vi "acquire single wave subvi.vi"(8 "error in (no error)":errorcluster, 10 "read buffer 5":string, 11 "VISA Refnum in":refnum<visa-resource-name>) -> (0 "Enum":enum16{"Idle", "Start"}(ring), 1 "String":string, 2 "read buffer":string, 3 "read buffer 3":string, 4 "Array":i32[](array[numeric]), 5 "read buffer 2":string, 6 "read buffer 6":string, 7 "read buffer 4":string)   [LabVIEW 2013]
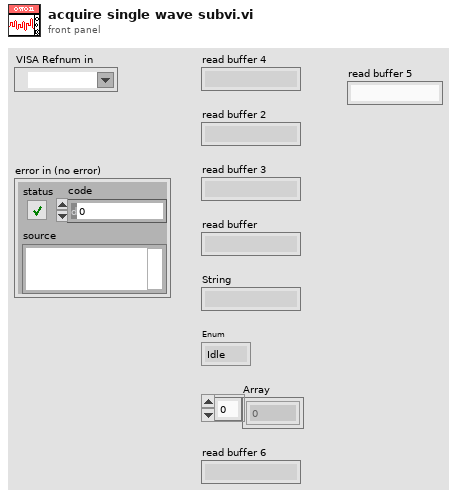
[diagram p1: front panel]
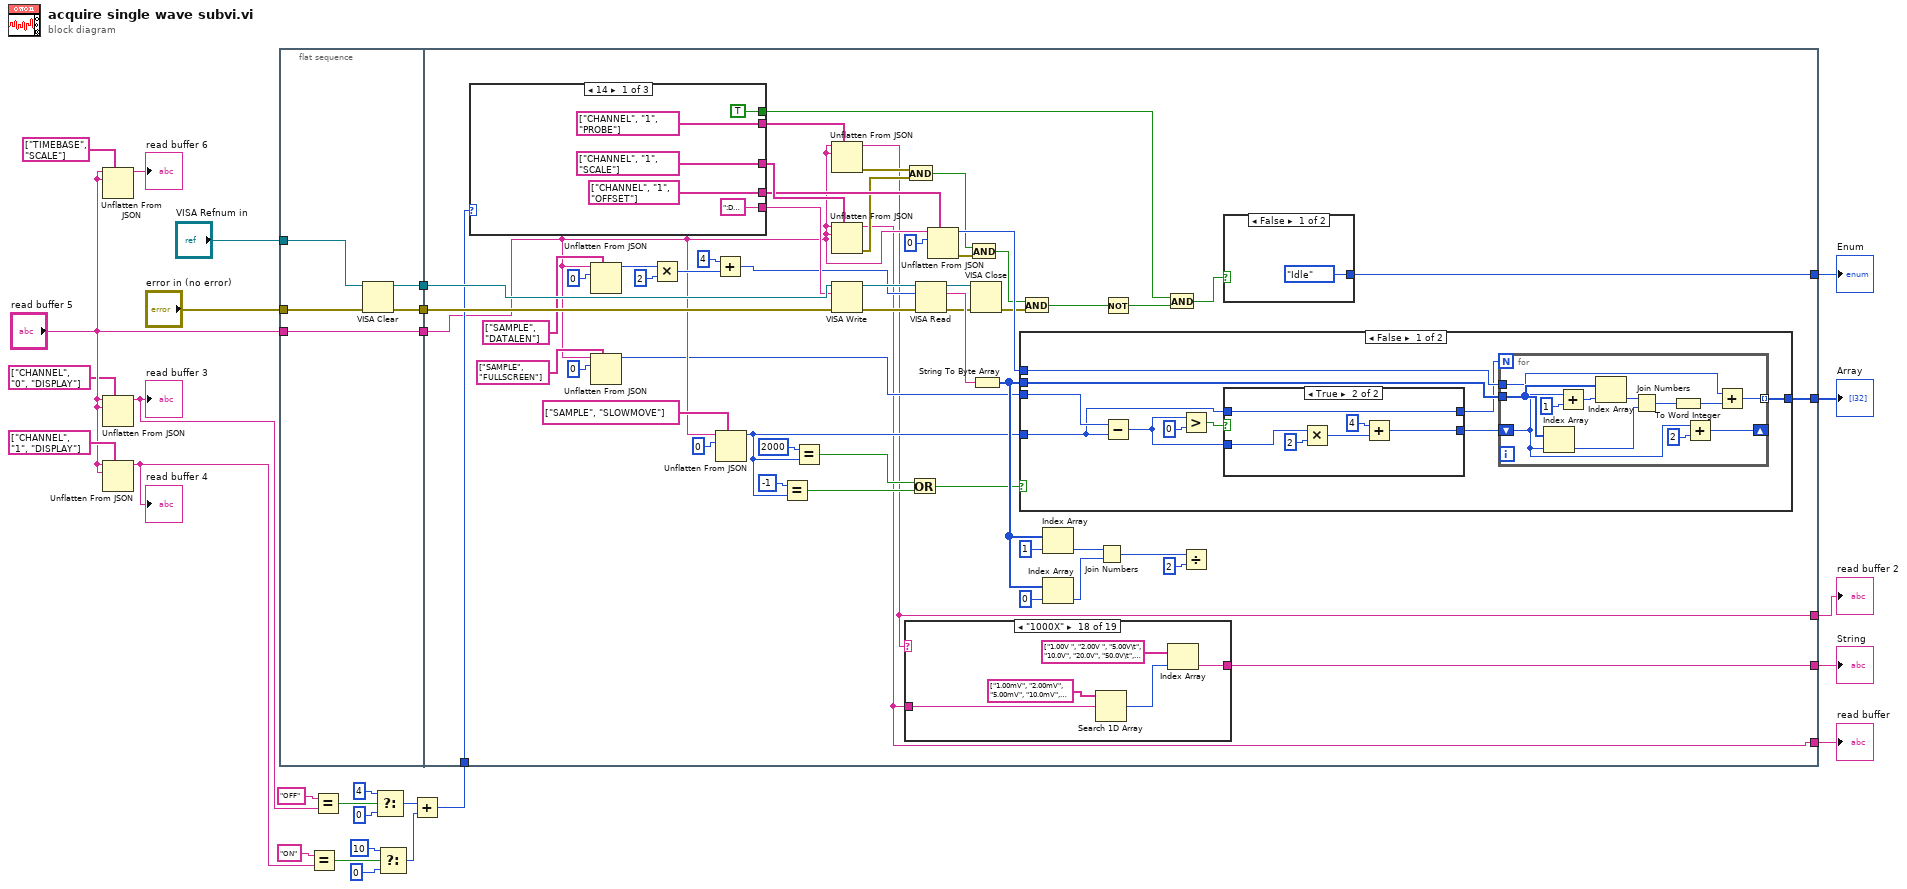
[diagram p0: block diagram]
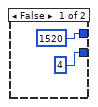
[diagram p2: hidden frame]
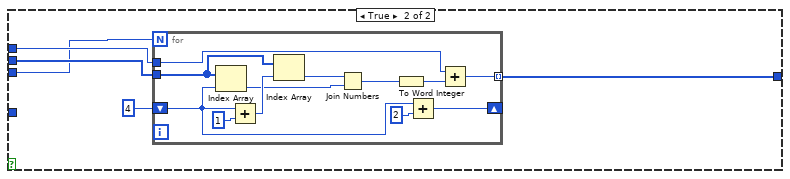
[diagram p3: hidden frame]
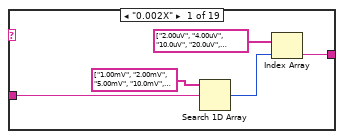
[diagram p4: hidden frame]
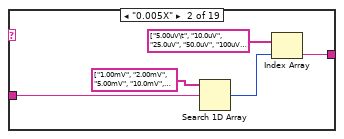
[diagram p5: hidden frame]
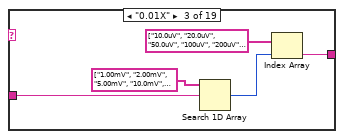
[diagram p6: hidden frame]
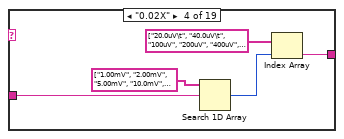
[diagram p7: hidden frame]
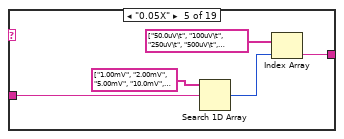
[diagram p8: hidden frame]
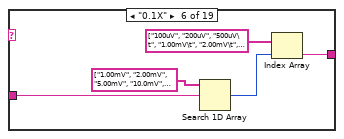
[diagram p9: hidden frame]
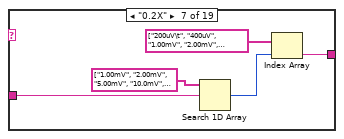
[diagram p10: hidden frame]
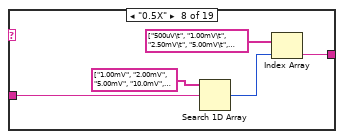
[diagram p11: hidden frame]
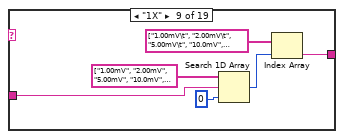
[diagram p12: hidden frame]
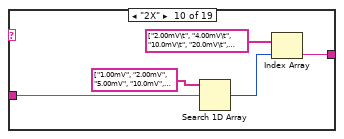
[diagram p13: hidden frame]
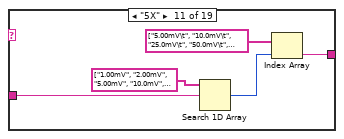
[diagram p14: hidden frame]
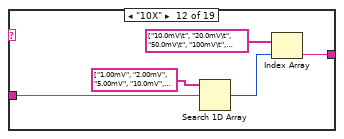
[diagram p15: hidden frame]
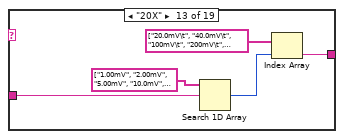
[diagram p16: hidden frame]
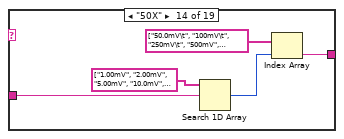
[diagram p17: hidden frame]
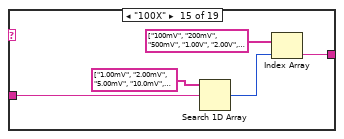
[diagram p18: hidden frame]
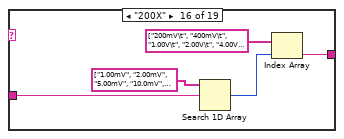
[diagram p19: hidden frame]
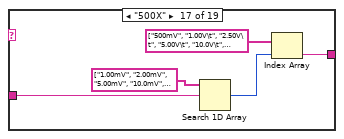
[diagram p20: hidden frame]
diagram:
  n1 = Unflatten From JSON(path=string[] ["TIMEBASE", "SCALE"], JSON string="read buffer 5", type and defaults="read buffer 5") -> (value=→"read buffer 6":string)  [unwired: 4 in, 1 out]
  n2 = Unflatten From JSON(path=string[] ["CHANNEL", "0", "DISPLAY"], JSON string="read buffer 5", type and defaults="read buffer 5") -> (value=w11:string)  [unwired: 4 in, 1 out]
  "read buffer 3" <- w11
  n3 = Unflatten From JSON(path=string[] ["CHANNEL", "1", "DISPLAY"], JSON string="read buffer 5", type and defaults="read buffer 5") -> (value=w9:string)  [unwired: 4 in, 1 out]
  "read buffer 4" <- w9
  n4 = flat-sequence {
    tunnel: "read buffer 5" -> [w33]
    tunnel: [w32] -> w28
    tunnel: [w31] -> w27
    tunnel: [w33] -> w26
    tunnel: "VISA Refnum in" -> [w30]
    tunnel: "error in (no error)" -> [w29]
    tunnel: [w70] -> w6
    tunnel: w28 -> [w88]
    tunnel: w27 -> [w87]
    tunnel: w26 -> [w45]
    tunnel: w21 -> [w60]
    tunnel: [w37] -> w22
    tunnel: [w36] -> w23
    tunnel: [w35] -> w24
    tunnel: [w34] -> w25
    frame #0 {
      n5 = VISA Clear(VISA resource name=w30, error in (no error)=w29) -> (VISA resource name out=w32:refnum<visa-resource-name>, error out=w31:errorcluster)
    }
    frame #1 {
      n6 = case shown="14" w60 {
        tunnel: [":DATA:WAVE:SCREEN:CH2?" ("ID Query") _ ":DATA:WAVE:SCREEN:CH1?" ("ID Query")] -> w84
        tunnel: [string[] ["CHANNEL", "1", "PROBE"] _ string[] ["CHANNEL", "0", "PROBE"]] -> w78
        tunnel: [string[] ["CHANNEL", "1", "SCALE"] _ string[] ["CHANNEL", "0", "SCALE"]] -> w77
        tunnel: [string[] ["CHANNEL", "1", "OFFSET"] _ string[] ["CHANNEL", "0", "OFFSET"]] -> w73
        tunnel: [TRUE FALSE TRUE] -> w59
        frame 14 {
        }
        frame 4, Default {
          n7 = call "显示对话框信息"() -> ()  [unwired: 10 in, 2 out]
        }
        frame 0 {
        }
      }
      n8 = Unflatten From JSON(path=string[] ["SAMPLE", "DATALEN"], JSON string=w45, type and defaults=0) -> (value=w67:i32)  [unwired: 4 in, 1 out]
      n9 = Unflatten From JSON(path=string[] ["SAMPLE", "FULLSCREEN"], JSON string=w45, type and defaults=0) -> (value=w44:i32)  [unwired: 4 in, 1 out]
      n10 = Multiply(x=w67, y=2) -> (x*y=w65:i32)
      n11 = Add(x=4, y=w65) -> (x+y=w61:i32)
      n12 = Unflatten From JSON(path=string[] ["SAMPLE", "SLOWMOVE"], JSON string=w45, type and defaults=0) -> (value=w38:i32)  [unwired: 4 in, 1 out]
      n13 = Equal?(x=-1, y=w38) -> (x = y?=w41:bool)
      n14 = Equal?(x=2000, y=w38) -> (x = y?=w40:bool)
      n15 = Unflatten From JSON(path=w78, JSON string=w45, type and defaults=w45) -> (value=w35:string, error out=w56:errorcluster)  [unwired: 4 in]
      n16 = Unflatten From JSON(path=w77, JSON string=w45, type and defaults=w45) -> (value=w34:string, error out=w55:errorcluster)  [unwired: 4 in]
      n17 = VISA Write(VISA resource name=w88, write buffer=w84, error in (no error)=w87) -> (VISA resource name out=w86:refnum<visa-resource-name>, error out=w85:errorcluster)  [unwired: 1 out]
      n18 = case shown="\"1000X\"" w35 {
        tunnel: w34 -> [w139 w144 w149 w154 w159 w164 w169 w174 w179 w185 w190 w195 w200 w205 w210 w215 w220 w225 w231]
        tunnel: [w138 w143 w148 w153 w158 w163 w168 w173 w178 w184 w189 w194 w199 w204 w209 w214 w219 w224 w228] -> w36
        frame "0.002X" {
          n19 = Search 1D Array(1D array=string[] ["1.00mV", "2.00mV", "5.00mV", "10.0mV", "20.0mV", "50.0mV", "100mV", "200mV", "500mV", "1.00V", "2.00V", "5.00V", "10.0V", "20.0V"], element=w139) -> (index of element=w140:i32)  [unwired: 1 in]
          n20 = Index Array(array=string[] ["2.00uV", "4.00uV", "10.0uV", "20.0uV", "50.0uV", "100uV", "200uV", "400uV", "1.00mV", "2.00mV\t", "4.00mV", "10.0mV", "20.0mV", "40.0mV"], index=w140) -> (element=w138:string)
        }
        frame "0.005X" {
          n21 = Search 1D Array(1D array=string[] ["1.00mV", "2.00mV", "5.00mV", "10.0mV", "20.0mV", "50.0mV", "100mV", "200mV", "500mV", "1.00V", "2.00V", "5.00V", "10.0V", "20.0V"], element=w144) -> (index of element=w145:i32)  [unwired: 1 in]
          n22 = Index Array(array=string[] ["5.00uV\t", "10.0uV", "25.0uV", "50.0uV", "100uV", "250uV", "500uV", "1.00mV\t", "2.50mV", "5.00mV", "10.0mV", "25.0mV", "50.0mV", "100mV"], index=w145) -> (element=w143:string)
        }
        frame "0.01X" {
          n23 = Search 1D Array(1D array=string[] ["1.00mV", "2.00mV", "5.00mV", "10.0mV", "20.0mV", "50.0mV", "100mV", "200mV", "500mV", "1.00V", "2.00V", "5.00V", "10.0V", "20.0V"], element=w149) -> (index of element=w150:i32)  [unwired: 1 in]
          n24 = Index Array(array=string[] ["10.0uV", "20.0uV", "50.0uV", "100uV", "200uV", "500uV", "1.00mV\t", "2.00mV\t", "5.00mV", "10.0mV\t", "20.0mV\t", "50.0mV", "100mV", "200mV"], index=w150) -> (element=w148:string)
        }
        frame "0.02X" {
          n25 = Search 1D Array(1D array=string[] ["1.00mV", "2.00mV", "5.00mV", "10.0mV", "20.0mV", "50.0mV", "100mV", "200mV", "500mV", "1.00V", "2.00V", "5.00V", "10.0V", "20.0V"], element=w154) -> (index of element=w155:i32)  [unwired: 1 in]
          n26 = Index Array(array=string[] ["20.0uV\t", "40.0uV\t", "100uV", "200uV", "400uV", "1.00mV", "2.00mV", "4.00mV", "10.0mV", "20.0mV", "40.0mV", "100mV", "200mV", "400mV"], index=w155) -> (element=w153:string)
        }
        frame "0.05X" {
          n27 = Search 1D Array(1D array=string[] ["1.00mV", "2.00mV", "5.00mV", "10.0mV", "20.0mV", "50.0mV", "100mV", "200mV", "500mV", "1.00V", "2.00V", "5.00V", "10.0V", "20.0V"], element=w159) -> (index of element=w160:i32)  [unwired: 1 in]
          n28 = Index Array(array=string[] ["50.0uV\t", "100uV\t", "250uV\t", "500uV\t", "1.00mV", "2.50mV\t", "5.00mV\t", "10.0mV\t", "25.0mV", "50.0mV\t", "100mV", "250mV", "500mV", "1.00V"], index=w160) -> (element=w158:string)
        }
        frame "0.1X" {
          n29 = Search 1D Array(1D array=string[] ["1.00mV", "2.00mV", "5.00mV", "10.0mV", "20.0mV", "50.0mV", "100mV", "200mV", "500mV", "1.00V", "2.00V", "5.00V", "10.0V", "20.0V"], element=w164) -> (index of element=w165:i32)  [unwired: 1 in]
          n30 = Index Array(array=string[] ["100uV", "200uV", "500uV\t", "1.00mV\t", "2.00mV\t", "5.00mV\t", "10.0mV\t", "20.0mV\t", "50.0mV\t", "100mV", "200mV", "500mV\t", "1.00V", "2.00V"], index=w165) -> (element=w163:string)
        }
        frame "0.2X" {
          n31 = Search 1D Array(1D array=string[] ["1.00mV", "2.00mV", "5.00mV", "10.0mV", "20.0mV", "50.0mV", "100mV", "200mV", "500mV", "1.00V", "2.00V", "5.00V", "10.0V", "20.0V"], element=w169) -> (index of element=w170:i32)  [unwired: 1 in]
          n32 = Index Array(array=string[] ["200uV\t", "400uV", "1.00mV", "2.00mV", "4.00mV\t", "10.0mV", "20.0mV", "40.0mV\t", "100mV", "200mV", "400mV", "1.00V", "2.00V", "4.00V"], index=w170) -> (element=w168:string)
        }
        frame "0.5X" {
          n33 = Search 1D Array(1D array=string[] ["1.00mV", "2.00mV", "5.00mV", "10.0mV", "20.0mV", "50.0mV", "100mV", "200mV", "500mV", "1.00V", "2.00V", "5.00V", "10.0V", "20.0V"], element=w174) -> (index of element=w175:i32)  [unwired: 1 in]
          n34 = Index Array(array=string[] ["500uV\t", "1.00mV\t", "2.50mV\t", "5.00mV\t", "10.0mV\t", "25.0mV\t", "50.0mV\t", "100mV", "250mV\t", "500mV\t", "1.00V\t", "2.50V\t", "5.00V\t", "10.0V"], index=w175) -> (element=w173:string)
        }
        frame "1X" {
          n35 = Search 1D Array(1D array=string[] ["1.00mV", "2.00mV", "5.00mV", "10.0mV", "20.0mV", "50.0mV", "100mV", "200mV", "500mV", "1.00V", "2.00V", "5.00V", "10.0V", "20.0V"], element=w179, start index (0)=0 ("开始索引(0)")) -> (index of element=w180:i32)
          n36 = Index Array(array=string[] ["1.00mV\t", "2.00mV\t", "5.00mV\t", "10.0mV", "20.0mV", "50.0mV", "100mV", "200mV\t", "500mV", "1.00V\t", "2.00V", "5.00V", "10.0V", "20.0V"], index=w180) -> (element=w178:string)
        }
        frame "2X" {
          n37 = Search 1D Array(1D array=string[] ["1.00mV", "2.00mV", "5.00mV", "10.0mV", "20.0mV", "50.0mV", "100mV", "200mV", "500mV", "1.00V", "2.00V", "5.00V", "10.0V", "20.0V"], element=w185) -> (index of element=w186:i32)  [unwired: 1 in]
          n38 = Index Array(array=string[] ["2.00mV\t", "4.00mV\t", "10.0mV\t", "20.0mV\t", "40.0mV", "100mV\t", "200mV", "400mV", "1.00V\t", "2.00V", "4.00V", "10.0V", "20.0V", "40.0V"], index=w186) -> (element=w184:string)
        }
        frame "5X" {
          n39 = Search 1D Array(1D array=string[] ["1.00mV", "2.00mV", "5.00mV", "10.0mV", "20.0mV", "50.0mV", "100mV", "200mV", "500mV", "1.00V", "2.00V", "5.00V", "10.0V", "20.0V"], element=w190) -> (index of element=w191:i32)  [unwired: 1 in]
          n40 = Index Array(array=string[] ["5.00mV\t", "10.0mV\t", "25.0mV\t", "50.0mV\t", "100mV\t", "250mV\t", "500mV", "1.00V", "2.50V\t", "5.00V", "10.0V\t", "25.0V", "50.0V ", "100V"], index=w191) -> (element=w189:string)
        }
        frame "10X" {
          n41 = Search 1D Array(1D array=string[] ["1.00mV", "2.00mV", "5.00mV", "10.0mV", "20.0mV", "50.0mV", "100mV", "200mV", "500mV", "1.00V", "2.00V", "5.00V", "10.0V", "20.0V"], element=w195) -> (index of element=w196:i32)  [unwired: 1 in]
          n42 = Index Array(array=string[] ["10.0mV\t", "20.0mV\t", "50.0mV\t", "100mV\t", "200mV", "500mV\t", "1.00V", "2.00V\t", "5.00V\t", "10.0V\t", "20.0V\t", "50.0V", "100V ", "200V"], index=w196) -> (element=w194:string)
        }
        frame "20X" {
          n43 = Search 1D Array(1D array=string[] ["1.00mV", "2.00mV", "5.00mV", "10.0mV", "20.0mV", "50.0mV", "100mV", "200mV", "500mV", "1.00V", "2.00V", "5.00V", "10.0V", "20.0V"], element=w200) -> (index of element=w201:i32)  [unwired: 1 in]
          n44 = Index Array(array=string[] ["20.0mV\t", "40.0mV\t", "100mV\t", "200mV\t", "400mV", "1.00V\t", "2.00V\t", "4.00V\t", "10.0V\t", "20.0V\t", "40.0V", "100V", "200V\t", "400V"], index=w201) -> (element=w199:string)
        }
        frame "50X" {
          n45 = Search 1D Array(1D array=string[] ["1.00mV", "2.00mV", "5.00mV", "10.0mV", "20.0mV", "50.0mV", "100mV", "200mV", "500mV", "1.00V", "2.00V", "5.00V", "10.0V", "20.0V"], element=w205) -> (index of element=w206:i32)  [unwired: 1 in]
          n46 = Index Array(array=string[] ["50.0mV\t", "100mV\t", "250mV\t", "500mV", "1.00V", "2.50V\t", "5.00V\t", "10.0V\t", "25.0V\t", "50.0V\t", "100V", "250V", "500V\t", "1.00kV"], index=w206) -> (element=w204:string)
        }
        frame "100X" {
          n47 = Search 1D Array(1D array=string[] ["1.00mV", "2.00mV", "5.00mV", "10.0mV", "20.0mV", "50.0mV", "100mV", "200mV", "500mV", "1.00V", "2.00V", "5.00V", "10.0V", "20.0V"], element=w210) -> (index of element=w211:i32)  [unwired: 1 in]
          n48 = Index Array(array=string[] ["100mV", "200mV", "500mV", "1.00V", "2.00V", "5.00V", "10.0V", "20.0V", "50.0V", "100V   ", "200V", "500V", "1.00kV\t", "2.00kV"], index=w211) -> (element=w209:string)
        }
        frame "200X" {
          n49 = Search 1D Array(1D array=string[] ["1.00mV", "2.00mV", "5.00mV", "10.0mV", "20.0mV", "50.0mV", "100mV", "200mV", "500mV", "1.00V", "2.00V", "5.00V", "10.0V", "20.0V"], element=w215) -> (index of element=w216:i32)  [unwired: 1 in]
          n50 = Index Array(array=string[] ["200mV\t", "400mV\t", "1.00V\t", "2.00V\t", "4.00V\t", "10.0V\t", "20.0V\t", "40.0V\t", "100V   ", "200V    ", "400V   ", "1.00kV", "2.00kV", "4.00kV"], index=w216) -> (element=w214:string)
        }
        frame "500X" {
          n51 = Search 1D Array(1D array=string[] ["1.00mV", "2.00mV", "5.00mV", "10.0mV", "20.0mV", "50.0mV", "100mV", "200mV", "500mV", "1.00V", "2.00V", "5.00V", "10.0V", "20.0V"], element=w220) -> (index of element=w221:i32)  [unwired: 1 in]
          n52 = Index Array(array=string[] ["500mV", "1.00V\t", "2.50V\t", "5.00V\t", "10.0V\t", "25.0V", "50.0V", "100V   ", "250V\t", "500V\t    ", "1.00kV\t", "2.50kV", "5.00kV", "10.0kV"], index=w221) -> (element=w219:string)
        }
        frame "1000X" {
          n53 = Search 1D Array(1D array=string[] ["1.00mV", "2.00mV", "5.00mV", "10.0mV", "20.0mV", "50.0mV", "100mV", "200mV", "500mV", "1.00V", "2.00V", "5.00V", "10.0V", "20.0V"], element=w225) -> (index of element=w226:i32)  [unwired: 1 in]
          n54 = Index Array(array=string[] ["1.00V ", "2.00V ", "5.00V\t", "10.0V", "20.0V", "50.0V\t", "100V", "200V  ", "500V   ", "1.00kV\t   ", "2.00kV ", "5.00kV\t", "10.0kV", "20.0kV"], index=w226) -> (element=w224:string)
        }
        frame "0.001X", Default {
          n55 = Search 1D Array(1D array=string[] ["1.00mV", "2.00mV", "5.00mV", "10.0mV", "20.0mV", "50.0mV", "100mV", "200mV", "500mV", "1.00V", "2.00V", "5.00V", "10.0V", "20.0V"], element=w231) -> (index of element=w230:i32)  [unwired: 1 in]
          n56 = Index Array(array=string[] ["1.00uV", "2.00uV", "5.00uV", "10.0uV", "20.0uV", "50.0uV,\t", "100uV,\t", "200uV,\t", "500uV,\t", "1.00mV,\t", "2.00mV,\t", "5.00mV,\t", "10.0mV, ", "20.0mv"], index=w230) -> (element=w228:string)
        }
      }
      n57 = And(x=w56, y=w55) -> (x .and. y?=w53:bool)
      n58 = Or(x=w40, y=w41) -> (x .or. y?=w39:bool)
      n59 = VISA Read(VISA resource name=w86, byte count=w61, error in (no error)=w85) -> (VISA resource name out=w62:refnum<visa-resource-name>, read buffer=w79:string, error out=w63:errorcluster)  [unwired: 1 out]
      n60 = Unflatten From JSON(path=w73, JSON string=w45, type and defaults=0) -> (value=w71:i32, error out=w54:errorcluster)  [unwired: 4 in]
      n61 = And(x=w53, y=w54) -> (x .and. y?=w51:bool)
      n62 = VISA Close(VISA resource name=w62, error in (no error)=w63) -> (error out=w52:errorcluster)
      n63 = String To Byte Array(string=w79) -> (unsigned byte array=w76:u8[])
      n64 = case shown="False" w39 {
        tunnel: w76 -> [w96 w123]
        tunnel: w71 -> [w97 w121]
        tunnel: [w98 w120] -> w37
        tunnel: w44 -> [w95 w119]
        tunnel: w38 -> [w89 _]
        frame False {
          n65 = Subtract(x=w95, y=w89) -> (x-y=w92:i32)
          n66 = Greater?(x=w92, y=0) -> (0:w93:bool)
          n67 = case shown="True" w93 {
            tunnel: [4 w105] -> w94
            tunnel: w92 -> [_ w102]
            tunnel: [1520 w101] -> w90
            tunnel: w89 -> [_ w101]
            frame False {
            }
            frame True {
              n68 = Multiply(x=w102, y=2) -> (x*y=w104:i32)
              n69 = Add(x=4, y=w104) -> (x+y=w105:i32)
            }
          }
          n70 = for {
            N: w90 -> [_]
            tunnel: w96 -> [w118]
            shift-right: [w115] -> _
            shift-left: w94 -> [w114]
            tunnel: [w112] -> w98 mode=indexing
            tunnel: w97 -> [w109]
            n71 = Index Array(array=w118, index=w114) -> (element=w110:u8)
            n72 = Add(x=w114, y=1) -> (x+y=w117:i32)
            n73 = Index Array(array=w118, index=w117) -> (element=w111:u8)
            n74 = Join Numbers(hi=w111, lo=w110) -> ((hi.lo)=w108:u16)
            n75 = To Word Integer(number=w108) -> (16bit integer=w107:i16)
            n76 = Add(x=w114, y=2) -> (x+y=w115:i32)
            n77 = Add(x=w109, y=w107) -> (x+y=w112:i32)
          }
        }
        frame True {
          n78 = for {
            N: w119 -> [_]
            tunnel: w123 -> [w135]
            shift-right: [w132] -> _
            shift-left: 4 -> [w131]
            tunnel: [w129] -> w120 mode=indexing
            tunnel: w121 -> [w126]
            n79 = Index Array(array=w135, index=w131) -> (element=w127:u8)
            n80 = Add(x=w131, y=1) -> (x+y=w134:i32)
            n81 = Index Array(array=w135, index=w134) -> (element=w128:u8)
            n82 = Join Numbers(hi=w128, lo=w127) -> ((hi.lo)=w125:u16)
            n83 = To Word Integer(number=w125) -> (16bit integer=w124:i16)
            n84 = Add(x=w131, y=2) -> (x+y=w132:i32)
            n85 = Add(x=w126, y=w124) -> (x+y=w129:i32)
          }
        }
      }
      n86 = And(x=w51, y=w52) -> (x .and. y?=w50:bool)
      n87 = Index Array(array=w76, index=1) -> (element=w81:u8)
      n88 = Index Array(array=w76, index=0) -> (element=w80:u8)
      n89 = Join Numbers(hi=w81, lo=w80) -> ((hi.lo)=w75:u16)
      n90 = Not(x=w50) -> (.not. x?=w57:bool)
      n91 = And(x=w59, y=w57) -> (x .and. y?=w58:bool)
      n92 = Divide(x=w75, y=u16 2) -> ()  [unwired: 1 out]
      n93 = case shown="False" w58 {
        tunnel: [enum16{"Idle", "Start"}."Idle" enum16{"Idle", "Start"}."Start"] -> w70
        frame False {
        }
        frame True {
        }
      }
    }
  }
  n94 = Equal?(x="ON", y=w9) -> (x = y?=w13:bool)
  n95 = Equal?(x="OFF", y=w11) -> (x = y?=w14:bool)
  n96 = Select(t=4 ("offset (0)"), s=w14, f=0 ("offset (0)")) -> (s? t:f=w19:i32)
  n97 = Select(t=10 ("offset (0)"), s=w13, f=0 ("offset (0)")) -> (s? t:f=w20:i32)
  n98 = Add(x=w19, y=w20) -> (x+y=w21:i32)
  "read buffer" <- w25
  "read buffer 2" <- w24
  "String" <- w23
  "Array" <- w22
  "Enum" <- w6
